vi "Init_New.vi"(8 "error in (no error)":errorcluster, 11 "Instruments in":refnum<class "Instruments.lvclass">) -> (0 "error out":errorcluster, 3 "Instruments out":refnum<class "Instruments.lvclass">)   [LabVIEW 2012, in "Instruments.lvclass"]
uses:
  Instruments.lvclass
  Instruments.lvclass/Instruments.ctl
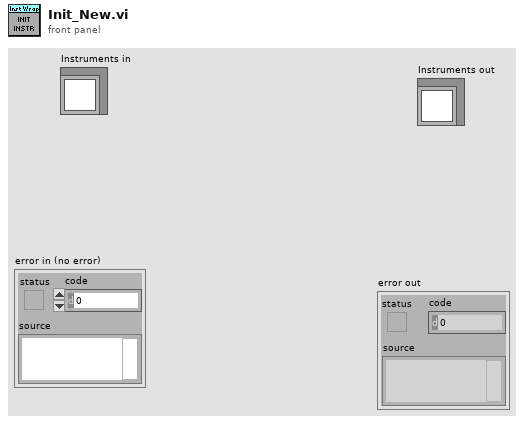
[diagram p1: front panel]
types:
  T1 = typedef "USB4000_Data.ctl" = cluster{"Wrapper Out":u32, "Number of Spectrometers":i32, "Wavelength":dbl[], "EL Spectrum":dbl[], "Int Time (usec)":i32, bool, "Background":dbl[]}
  T2 = typedef "Config.ctl" = cluster{"IntTime":i32, "Samples":i32, "PowerMin":dbl, "KneeMin":dbl, "KneeMax":dbl, "BackgroundWl":dbl}
  T3 = cluster{"Keithley_Param":cluster{"Start Current,mA":dbl, "Stop Current,mA":dbl, "Voltage Compliance,V":dbl, "GPIB":string}, "USB4000_Param":cluster{"Integration Time":i32, "Wl min,nm":dbl, "Wl max,nm":dbl, "USB4000":T1}, "Ophir_Param":cluster{"VISA resource name":refnum<visa-resource-name>, "Calibration Wl":dbl}, "Config":T2}
  T4 = cluster{"Start Current,mA":dbl, "Stop Current,mA":dbl, "Voltage Compliance,V":dbl, "GPIB":string}
  T5 = cluster{"error":bool, "code":i32, "source":string}
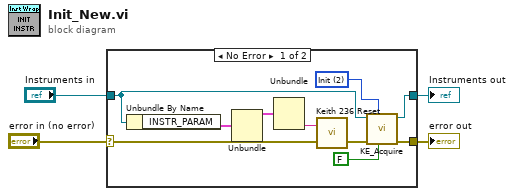
[diagram p0: block diagram]
diagram:
  n1 = case shown="No Error" "error in (no error)" {
    selector: "error in (no error)" -> [w11 w16]
    tunnel: [w7 w16] -> w3
    tunnel: [w10 w15] -> w1
    tunnel: "Instruments in" -> [w5 w15]
    frame No Error {
      w8 = u16 2 items=["First", "Second", "Init"] ("Type")
      n2 = Unbundle By Name(w5) -> ("INSTR_PARAM"=w12:T3)
      n3 = Unbundle(w12) -> ("Keithley_Param"=w13:T4)  [unwired: 3 out]
      n4 = Unbundle(w13) -> ("GPIB"=w14:string)  [unwired: 3 out]
      n5 = call "Keith 236 Reset.vi"("GPIB address"=w14, "error in"=w11) -> ("error out"=w6:T5)
      n6 = call-dynamic "KE_Acquire.vi"("KeepOn?"=FALSE ("Boolean"), "Type"=w8, "error in (no error)"=w6, "Instruments in"=w5) -> ("error out"=w7:errorcluster, "Instruments out"=w10:refnum<class "Instruments.lvclass">)  [unwired: 5 in, 1 out]
    }
    frame Error {
    }
  }
  "error out" <- w3
  "Instruments out" <- w1
